vi "ScreenCapture_test.vi"(1 "Height":u16, 2 "Width":u16, 3 "Folder-pass":path) -> ()   [LabVIEW 2018]
uses:
  System.Windows.Forms
  System.Drawing
panel:
  in  "PictureBox":refnum<k24>(container) caption="ピクチャボックス"
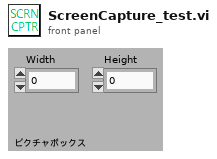
[diagram p1: front panel]
types:
  T1 = typedef "imagedata.ctl" = cluster{"image type":i32, "image depth":i32, "image":u8[], "mask":u8[], "colors":u32[], "Rectangle":cluster{"left":i16, "top":i16, "right":i16, "bottom":i16}}
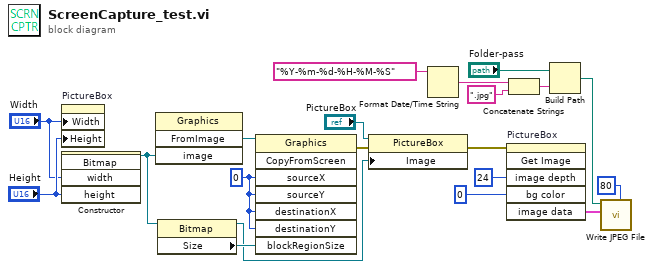
[diagram p0: block diagram]
diagram:
  w1 = 0 ("sourceX")
  n1 = property on="PictureBox" class="AXCont"("Width"="Width", "Height"="Height") -> ()  [unwired: 2 in, 2 out]
  n2 = constructor class="Bitmap"("width"="Width", "height"="Height") -> (reference out=w20:refnum<k24>)  [unwired: 3 in, 4 out]
  n3 = invoke class="Graphics" method="FromImage"("image"=w20) -> ("FromImage"=w18:refnum<k24>)  [unwired: 3 in, 3 out]
  n4 = property class="Bitmap"(reference=w20) -> (reference out=w2:refnum<k24>, "Size"=w17:refnum<k24>)  [unwired: 1 in, 1 out]
  n5 = invoke class="Graphics" method="CopyFromScreen"(reference=w18, "sourceX"=w1, "sourceY"=w1, "destinationX"=w1, "destinationY"=w1, "blockRegionSize"=w17) -> (error out=w19:errorcluster)  [unwired: 2 in, 7 out]
  n6 = property class="PictureBox"(reference="PictureBox", error in=w19, "Image"=w2) -> (error out=w5:errorcluster)  [unwired: 1 out]
  n7 = Format Date/Time String(time format string (%c)="%Y-%m-%d-%H-%M-%S") -> (date/time string=w7:string)  [unwired: 2 in]
  n8 = invoke on="PictureBox" class="AXCont" method="Get Image"(error in=w5, "image depth"=24 ("画像深度"), "bg color"=u32 0 ("背景色")) -> ("image data"=w13:T1)  [unwired: 3 in, 5 out]
  n9 = Concatenate Strings(w7, ".jpg") -> (w8:string)
  n10 = Build Path(base path="Folder-pass", name or relative path=w8) -> (appended path=w10:path)
  n11 = call <vilib>:"Write JPEG File.vi"("quality (80)"=80, "image data"=w13, "path to JPEG file"=w10) -> ()  [unwired: 7 in, 2 out]
